vi "RP Read Status TCP.vi"(6 "timeout ms (25000)":i32=1000, 8 "Error In":errorcluster, 9 "Status offset":u64, 10 "Read config":bool, 11 "connection ID":refnum<k5>) -> (0 "Error Out":errorcluster, 1 "Status response":u32=1 format="0x%x (%d)", 3 "connection ID out":refnum<k5>)   [LabVIEW 2019]
uses:
  RP Command.ctl
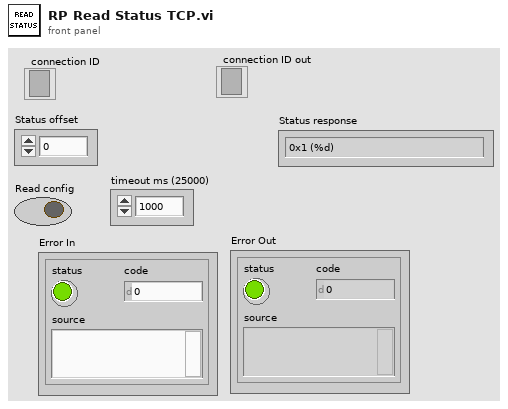
[diagram p1: front panel]
types:
  T1 = typedef "RP Command.ctl" = enum16{"Reset", "Read IDN", "Stop server", "Get status", "Get temperature", "Connect client", "Arm", "Software trigger", "Get whole buffer", "Get chunk", "System call", "Get config", "Set config", "Recieve data", "Recieve Calibartion", "Transmit data"}
  T2 = enum16{"big-endian, network order", "native, host order", "little-endian"}
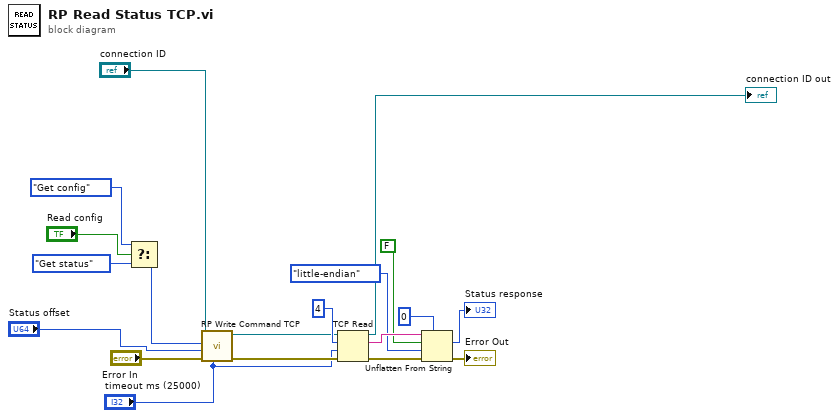
[diagram p0: block diagram]
diagram:
  n1 = Select(t=RP_Command."Get config" ("Command number"), s="Read config", f=RP_Command."Get status" ("Command number")) -> (s? t:f=w2:T1)
  n2 = call "RP Write Command TCP.vi"("timeout ms (25000)"="timeout ms (25000)", "Error In"="Error In", "Command payload"="Status offset", "Command number"=w2, "connection ID"="connection ID") -> ("Error Out"=w8:errorcluster, "connection ID out"=w9:refnum<k5>)  [unwired: 4 in, 1 out]
  n3 = TCP Read(connection ID=w9, bytes to read=4, error in (no error)=w8, 9:"timeout ms (25000)") -> (connection ID out=→"connection ID out":refnum<k5>, data out=w16:string, error out=w14:errorcluster)  [unwired: 1 in]
  n4 = Unflatten From String(type=u32 0, binary string=w16, data includes array or string size? (T)=FALSE, byte order (0:big-endian, network order)=T2."little-endian", error in (no error)=w14) -> (value=→"Status response":u32, error out=→"Error Out":errorcluster)  [unwired: 1 out]
